vi "Get Core Type.vi"(8 "error in (no error)":errorcluster, 11 "Instrument Owner in":refnum<class "Instrument Owner.lvclass">) -> (0 "error out":errorcluster, 3 "Sequencer Core out":refnum<class "Sequencer Core.lvclass">)   [LabVIEW 2020, in "Instrument Handler.lvlib" / "Instrument Owner.lvclass"]
doc: "Return the Sequencer Core type to launch with the Sequencer.\n\nThis implementation populates an Instrument Driver and adds it to the Instrument Sequencer that the VI returns."
uses:
  Instrument Owner.lvclass
  PPL/HDH.Actor Framework.Core.Sequencer.lvlibp/Sequencer Core/Sequencer Core.lvclass
  PPL/HDH.Actor Framework.Core.Instrument Driver.lvlibp/Instrument Driver/Instrument Driver.lvclass
  Instrument Owner.lvclass/Instrument Owner.ctl
  Instrument Sequencer/Instrument Sequencer.lvclass/Instrument Sequencer.ctl
  Instrument Sequencer/Instrument Sequencer.lvclass
  C:/Current projects/WS/PPL/HDH.Actor Framework.Core.Sequencer.lvlibp/Sequencer Core/Sequencer Core.lvclass
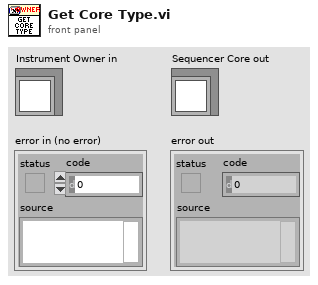
[diagram p1: front panel]
types:
  T1 = typedef "Instrument Handler.lvlib/Ctl_InstrumentSynchronicationCluster.ctl" = cluster{"Launched?":bool, "Driver Path":path, "Alias":string, "Connection Type":T2, "Pre Initialization Data":variant, "Enqueue Sync":refnum<class "Notifier.lvclass">, "Enqueue Lock":T3, "Owner Enqueuer":refnum<class "Message Enqueuer.lvclass">, "Owner":refnum<class "Sequencer Core.lvclass">, "Instrument ID":u32}
  T2 = typedef "HDH.Actor Framework.Core.Instrument Driver.lvlibp/Instrument Driver.lvclass/Ctl_ConnectionType.ctl" = enum16{"BuiltIn/System", "PXI/PCI", "USB", "GPIB", "VXI", "Serial", "TCP/IP", "cRIO", "SCXI", "cDAQ", "SwitchBlock", "SCC", "FireWire", "Accessory", "CAN", "SwitchBlock Device"}
  T3 = typedef "Semaphore RefNum" = refnum<k1>
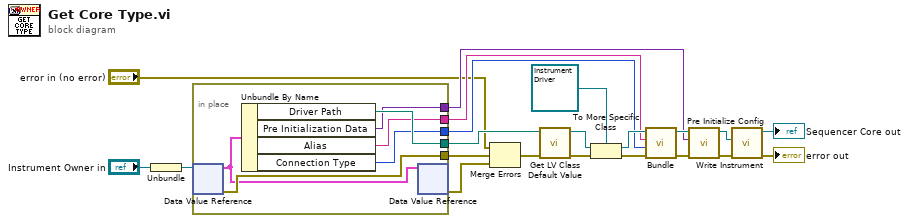
[diagram p0: block diagram]
diagram:
  n1 = Unbundle("Instrument Owner in") -> (w5:refnum<data-value>)
  n2 = in-place {
    in-place-border: [w27] -> w9
    in-place-border: [w26] -> w8
    in-place-border: [w25] -> w7
    in-place-border: [w24] -> w6
    in-place-border: [w23] -> w4
    n3 = in-place-dvr #1(w5) -> (w22:T1, w23:errorcluster)
    n4 = Unbundle By Name(w22) -> ("Driver Path"=w27:path, "Pre Initialization Data"=w26:variant, "Alias"=w25:string, "Connection Type"=w24:T2)
    n5 = in-place-dvr #1(w22) -> (w2:errorcluster)  [unwired: 1 out]
  }
  n6 = Merge Errors("error in (no error)", w4, w2) -> (w1:errorcluster)
  n7 = call <vilib>:"Get LV Class Default Value.vi"("error in (no error)"=w1, "class path"=w9) -> ("error out"=w19:errorcluster, "object"=w21:refnum<class>)  [unwired: 8 in]
  n8 = To More Specific Class(target class=refnum<class "Instrument Driver.lvclass"> refnum ("HDH.Actor Framework.Core.Instrument Driver.lvlibp:Instrument Driver.lvclass"), reference=w21, error in=w19) -> (specific class reference=w14:refnum<class "Instrument Driver.lvclass">, error out=w12:errorcluster)
  n9 = call "Bundle.vi"("error in (no error)"=w12, "Connection Type"=w6, "Alias"=w7, "Instrument in"=w14) -> ("error out"=w11:errorcluster, "Instrument out"=w13:refnum<class "Instrument Driver.lvclass">)  [unwired: 6 in]
  n10 = call-dynamic "Pre Initialize Config.vi"("error in (no error)"=w11, "Pre Initialization Data"=w8, "Instrument in"=w13) -> ("error out"=w15:errorcluster, "Instrument out"=w16:refnum<class "Instrument Driver.lvclass">)  [unwired: 6 in, 1 out]
  n11 = call "Write Instrument.vi"("error in (no error)"=w15, "Instrument Driver"=w16) -> ("error out"=→"error out":errorcluster, "Instrument Sequencer out"=→"Sequencer Core out":refnum<class "Instrument Sequencer.lvclass">)  [unwired: 8 in]
